vi "Delete_First_Rows.vi"(0 "File Type":string, 1 "Data In":string[][](array[string])) -> (2 "Rows removed":i32, 3 "Deleted Rows":string[][](array[string]), 4 "Data Out":string[][](array[string]))   [LabVIEW 2015]
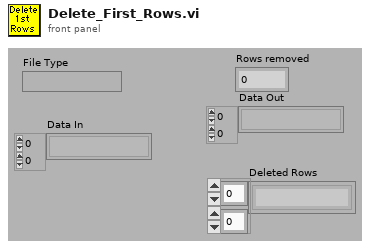
[diagram p1: front panel]
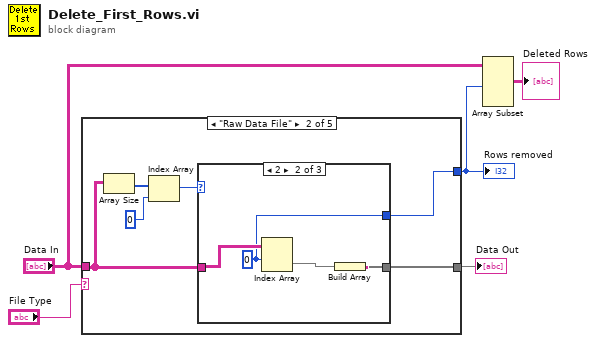
[diagram p0: block diagram]
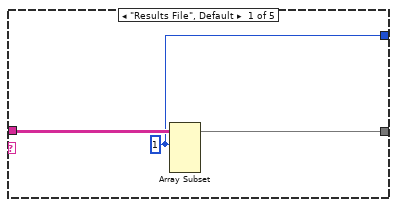
[diagram p2: hidden frame]
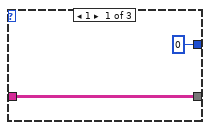
[diagram p3: hidden frame]
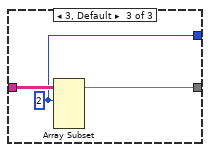
[diagram p4: hidden frame]
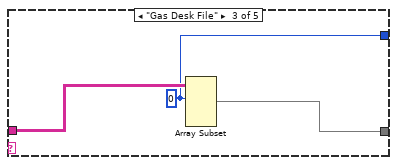
[diagram p5: hidden frame]
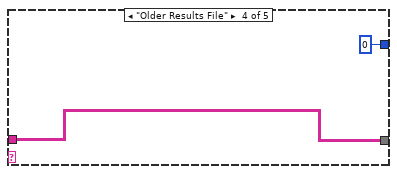
[diagram p6: hidden frame]
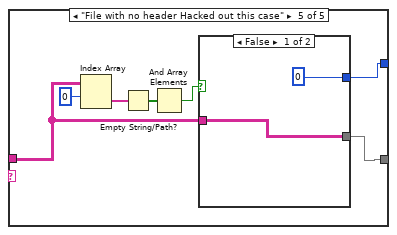
[diagram p7: hidden frame]
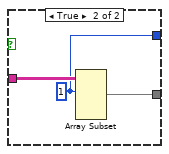
[diagram p8: hidden frame]
diagram:
  n1 = case shown="\"Raw Data File\"" "File Type" {
    tunnel: [w7 w14 w25 w28 w31] -> w5
    tunnel: "Data In" -> [w8 w12 w26 w28 w32]
    tunnel: [w6 w9 w24 0 ("Array Index") w29] -> w2
    frame "Results File", Default {
      w6 = 1 ("Array Index")
      n2 = Array Subset(array=w8, index (row)=w6) -> (w7:string[][])  [unwired: 3 in]
    }
    frame "Raw Data File" {
      n3 = Array Size(array=w12) -> (size(s)=w13:i32[])
      n4 = Index Array(array=w13, index=0 ("Index")) -> (element=w10:i32)
      n5 = case shown="2" w10 {
        tunnel: [w16 w18 w23] -> w14
        tunnel: w12 -> [w16 w20 w22]
        tunnel: [0 w17 w21] -> w9
        frame 1 {
        }
        frame 2 {
          w17 = 0 ("Index")
          n6 = Index Array(array=w20, index (row)=w17) -> (element=w19:string[])  [unwired: 1 in]
          n7 = Build Array(w19) -> (w18:string[][])
        }
        frame 3, Default {
          w21 = 2 ("Array Index")
          n8 = Array Subset(array=w22, index (row)=w21) -> (w23:string[][])  [unwired: 3 in]
        }
      }
    }
    frame "Gas Desk File" {
      w24 = 0 ("Array Index")
      n9 = Array Subset(array=w26, index (row)=w24) -> (w25:string[][])  [unwired: 3 in]
    }
    frame "Older Results File" {
    }
    frame "File with no header Hacked out this case" {
      n10 = Index Array(array=w32, index (row)=0) -> (element=w34:string[])  [unwired: 1 in]
      n11 = Empty String/Path?(string/path=w34) -> (empty?=w33:bool[])
      n12 = And Array Elements(Boolean array=w33) -> (logical AND=w30:bool)
      n13 = case shown="False" w30 {
        tunnel: w32 -> [w36 w40]
        tunnel: [w36 w39] -> w31
        tunnel: [0 ("Array Index") w38] -> w29
        frame False {
        }
        frame True {
          w38 = 1 ("Array Index")
          n14 = Array Subset(array=w40, index (row)=w38) -> (w39:string[][])  [unwired: 3 in]
        }
      }
    }
  }
  "Data Out" <- w5
  "Rows removed" <- w2
  n15 = Array Subset(array="Data In", length (row)=w2) -> (→"Deleted Rows":string[][])  [unwired: 3 in]
